vi "Logging Message Loop.vi"(8 "error in (no error)":errorcluster, 10 "Data Queue":refnum<queue>, 11 "Message Queues":T1) -> (0 "error out":errorcluster)   [LabVIEW 2014, in "Flicker.lvlib" / "Flicker Logging.lvlib"]
doc: "The message loop subVI to handle messages pertaining to logging data."
uses:
  Flicker Logging.lvlib
  support/Message Queue/All Message Queues.ctl
  support/Message Queue/Message Cluster.ctl
  Logging Configuration.ctl
  controls/Sphere Indicator.ctl
  controls/Metadata Cluster.ctl
  support/Message Queue/Enqueue Message (Single).vi
  <vilib>/Utility/error.llb/Error Cluster From Error Code.vi
  <vilib>/ErrorRing/Error Ring.xnode
  support/Message Queue/Flicker Message Queue.lvlib
  Flicker.lvlib
panel:
  in  "Stand alone?":bool=TRUE
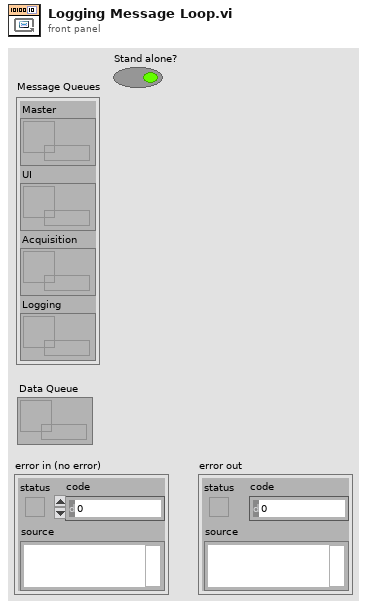
[diagram p1: front panel]
types:
  T1 = typedef "Flicker.lvlib/Flicker Message Queue.lvlib/All Message Queues.ctl" = cluster{"Master":refnum<queue>, "UI":refnum<queue>, "Acquisition":refnum<queue>, "Logging":refnum<queue>}
  T2 = typedef "Flicker.lvlib/Flicker Logging.lvlib/Logging Configuration.ctl" = cluster{"Log File Base Path":path, "TDMS File Reference":refnum<k34>}
  T3 = typedef "Flicker.lvlib/Sphere Indicator.ctl" = enum16{"Naked Sphere", "Insulated Sphere"}
  T4 = typedef "Flicker.lvlib/Metadata Cluster.ctl" = cluster{"Naked Sphere Metadata":string[][], "Insulated Sphere Metadata":string[][], "Output Path":path}
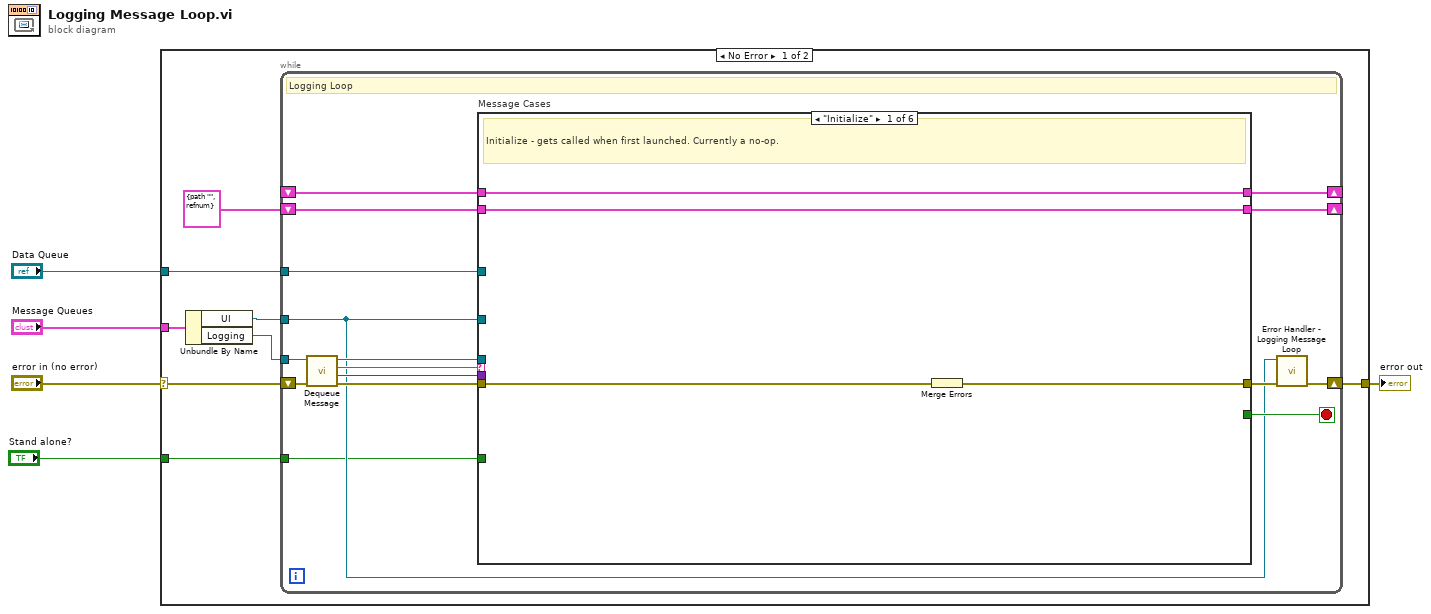
[diagram p0: block diagram]
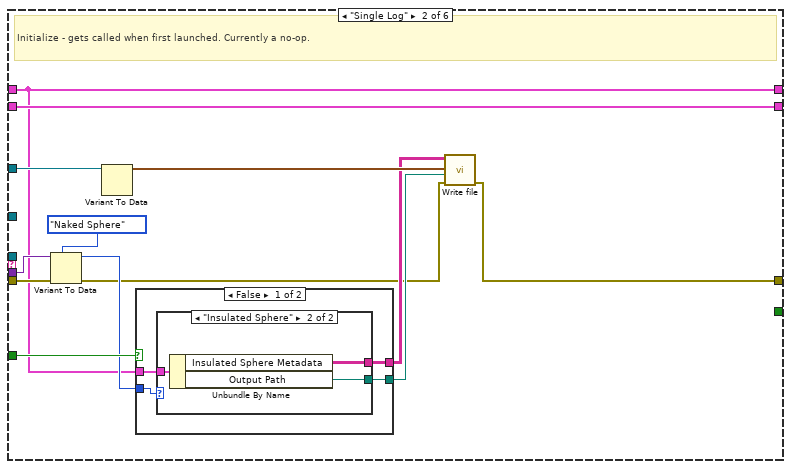
[diagram p2: hidden frame]
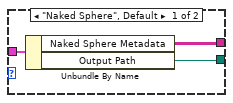
[diagram p3: hidden frame]
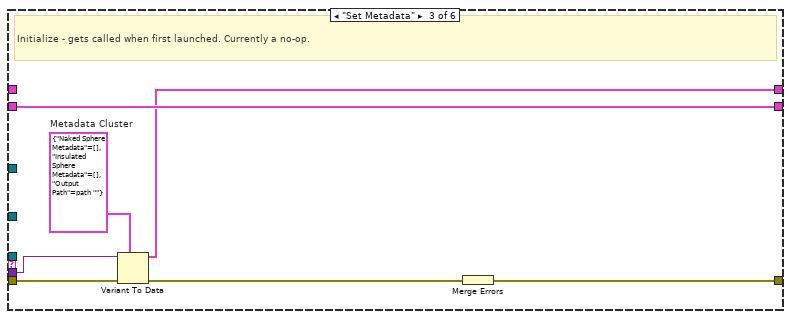
[diagram p5: hidden frame]
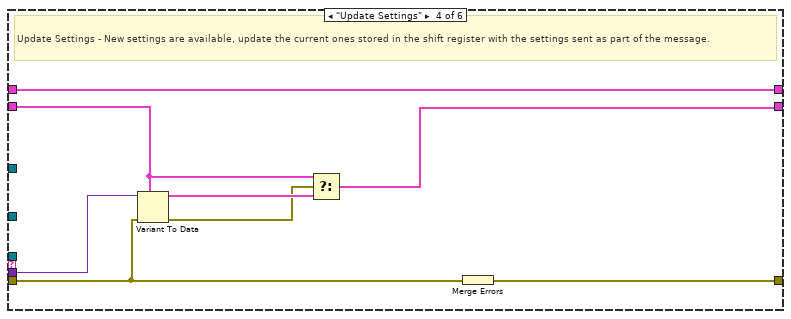
[diagram p6: hidden frame]
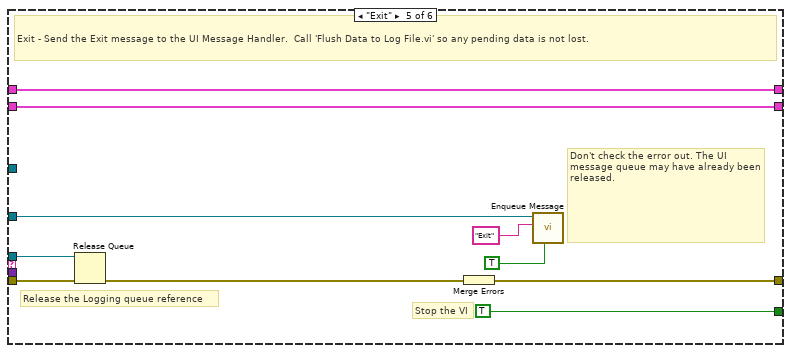
[diagram p7: hidden frame]
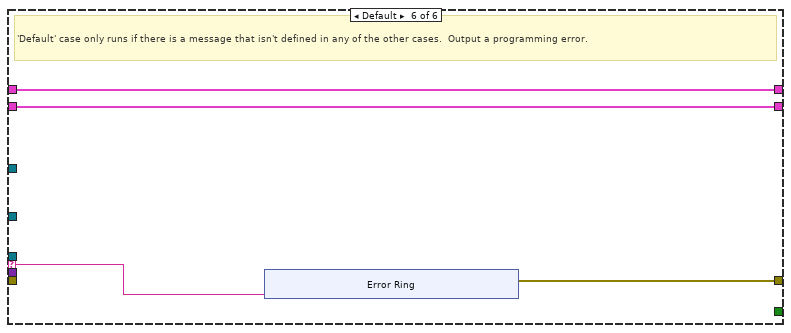
[diagram p8: hidden frame]
diagram:
  n1 = case shown="No Error" "error in (no error)" {
    selector: "error in (no error)" -> [w9 w93]
    tunnel: "Message Queues" -> [w13 _]
    tunnel: [w11 w93] -> w4
    tunnel: "Data Queue" -> [w8 _]
    tunnel: "Stand alone?" -> [w6 _]
    frame No Error {
      n2 = Unbundle By Name(w13) -> ("UI"=w7:refnum<queue>, "Logging"=w12:refnum<queue>)
      n3 = while {
        tunnel: w12 -> [w21]
        shift-right: [w28] -> _
        shift-left: T2 {"Log File Base Path"=path "", "TDMS File Reference"=refnum} ("Logging Configuration") -> [w29]
        shift-right: [w19] -> w11
        shift-left: w9 -> [w26]
        tunnel: w7 -> [w17]
        tunnel: w8 -> [w20]
        tunnel: w6 -> [w16]
        shift-right: [w15] -> _
        shift-left: _ -> [w14]
        stop <- w27 stop-if-true
        # "Logging Loop"
        n4 = call "Dequeue Message.vi"("error in (no error)"=w26, "Message Queue"=w21) -> ("error out"=w25:errorcluster, "Message Data"=w23:variant, "Message"=w24:string, "dup Message Queue"=w22:refnum<queue>)  [unwired: 6 in]
        n5 = case "Message Cases" shown="\"Initialize\"" w24 {
          selector: w24 -> [_ _ _ _ _ w83]
          tunnel: w22 -> [_ _ _ _ w75 _]
          tunnel: w25 -> [w31 w42 w61 w65 w78 _]
          tunnel: [w33 w34 w63 w71 w80 w84] -> w18
          tunnel: w29 -> [w32 w46 w62 w69 w73 w85]
          tunnel: [w32 w46 w62 w66 w73 w85] -> w28
          tunnel: [_ _ _ _ TRUE _] -> w27
          tunnel: w23 -> [_ w41 w59 w70 _ _]
          tunnel: w17 -> [_ _ _ _ w79 _]
          tunnel: w20 -> [_ w45 _ _ _ _]
          tunnel: w16 -> [_ w43 _ _ _ _]
          tunnel: [w30 w38 w57 w64 w72 w82] -> w15
          tunnel: w14 -> [w30 w38 _ w64 w72 w82]
          frame "Initialize" {
            # "Initialize - gets called when first launched. Currently a no-op."
            n6 = Merge Errors(w31) -> (w33:errorcluster)
          }
          frame "Single Log" {
            # "Initialize - gets called when first launched. Currently a no-op."
            n7 = Variant To Data(error in=w42, type=Sphere_Indicator."Naked Sphere" ("Sphere Indicator"), Variant=w41) -> (data=w39:T3, error out=w35:errorcluster)
            n8 = Variant To Data(Variant=w45) -> (data=w44:waveform(dbl))  [unwired: 2 in, 1 out]
            n9 = case shown="False" w43 {
              tunnel: w39 -> [w50 _]
              tunnel: w38 -> [w49 _]
              tunnel: [w48 _] -> w37
              tunnel: [w47 _] -> w36
              frame False {
                n10 = case shown="\"Insulated Sphere\"" w50 {
                  tunnel: w49 -> [w53 w56]
                  tunnel: [w52 w55] -> w48
                  tunnel: [w51 w54] -> w47
                  frame "Naked Sphere", Default {
                    n11 = Unbundle By Name(w53) -> ("Naked Sphere Metadata"=w52:string[][], "Output Path"=w51:path)
                  }
                  frame "Insulated Sphere" {
                    n12 = Unbundle By Name(w56) -> ("Insulated Sphere Metadata"=w55:string[][], "Output Path"=w54:path)
                  }
                }
              }
              frame True {
                # "feature to be added later"
              }
            }
            n13 = call "Write file.vi"("error in (no error)"=w35, "Logging Path"=w36, "Flicker Waveform"=w44, "Metadata"=w37) -> ("error out"=w34:errorcluster)  [unwired: 6 in, 1 out]
          }
          frame "Set Metadata" {
            w58 = T4 {"Naked Sphere Metadata"=[], "Insulated Sphere Metadata"=[], "Output Path"=path ""}  # Metadata Cluster
            # "Initialize - gets called when first launched. Currently a no-op."
            n14 = Variant To Data(error in=w61, type=w58, Variant=w59) -> (data=w57:T4, error out=w60:errorcluster)
            n15 = Merge Errors(w60) -> (w63:errorcluster)
          }
          frame "Update Settings" {
            # "Update Settings - New settings are available, update the current ones stored in the shift register with the settings sent as part of the message."
            n16 = Variant To Data(error in=w65, type=w69, Variant=w70) -> (data=w68:T2, error out=w67:errorcluster)
            n17 = Select(t=w69, s=w67, f=w68) -> (s? t:f=w66:T2)
            n18 = Merge Errors(w65) -> (w71:errorcluster)
          }
          frame "Exit" {
            # "Release the Logging queue reference"
            # "Don't check the error out. The UI message queue may have already been released."
            # "Stop the VI"
            # "Exit - Send the Exit message to the UI Message Handler.  Call 'Flush Data to Log File.vi' so any pending data is not lost."
            n19 = Release Queue(queue=w75, error in (no error)=w78) -> (error out=w74:errorcluster)  [unwired: 1 in, 2 out]
            n20 = Merge Errors(w74) -> (w80:errorcluster)
            n21 = call-poly "Enqueue Message.vi"("Priority Message? (F)"=TRUE, "Message"="Exit", "Message Queue"=w79) -> ()  [unwired: 7 in, 2 out]
          }
          frame Default {
            # "'Default' case only runs if there is a message that isn't defined in any of the other cases.  Output a programming error."
            n22 = xnode "Error Ring"("parameter 0"=w83) -> ("error out"=w84:errorcluster)
          }
        }
        n23 = call "Error Handler - Logging Message Loop.vi"("error in (no error)"=w18, "Message Queue"=w17) -> ("dup error in"=w19:errorcluster)  [unwired: 8 in, 1 out]
      }
    }
    frame Error {
    }
  }
  "error out" <- w4
